vi "Nyquist Shift.vi"(1 "X":dbl[](array[numeric]) format="%.2f") -> (0 "Nyquist Shift{X}":dbl[](array[numeric]) format="%.2f")   [LabVIEW 2009]
doc: "Subvi for DC Centered Spectrum.\n\nThis VI performs a conversion on a time domain sequence such that when the converted sequence is transformed to the frequency domain the result is the DC centered spectrum of the original time domain sequence."
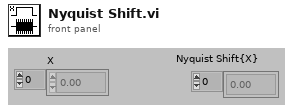
[diagram p1: front panel]
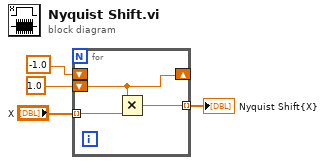
[diagram p0: block diagram]
diagram:
  n1 = for {
    shift-right: [w5] -> _
    shift-left: -1.0 -> [_]
    shift-left: 1.0 -> [w5]
    tunnel: "X" -> [w7] mode=indexing
    tunnel: [w6] -> w3 mode=indexing
    n2 = Multiply(x=w5, y=w7) -> (x*y=w6:dbl)
  }
  "Nyquist Shift{X}" <- w3
